vi "Calibrate_To_0.vi"(10 "Port":T2 items=["Port 1", "Port 2", "Port 3", "Port 4"], 11 "NXT":T1) -> (3 "NXT 2":T1)   [LabVIEW 2010]
uses:
  <vilib>/NXT/Subs/LVHSConnector.ctl
  <vilib>/NXT/Block Support/NXT_InputPort.ctl
  <vilib>/NXT/Dual Mode Library/Sensors/i2c_sensors.vi
panel:
  # "THIS FUNCTION WILL SIMPLY WRITE 0's TO ALL REGISTERS.\nTHIS ALLOWS MULTIPLE CALIBRATIONS WITHOUT POWERING DOWN."
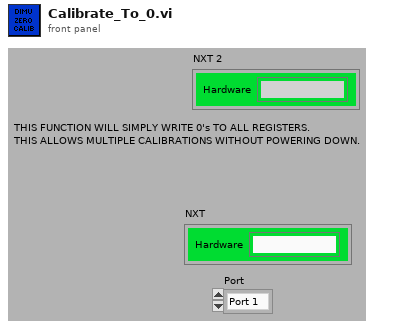
[diagram p1: front panel]
types:
  T1 = typedef "LVHSConnector.ctl" = cluster{"Hardware":string, "Flattened String":string}
  T2 = typedef "NXT_InputPort.ctl" = u8
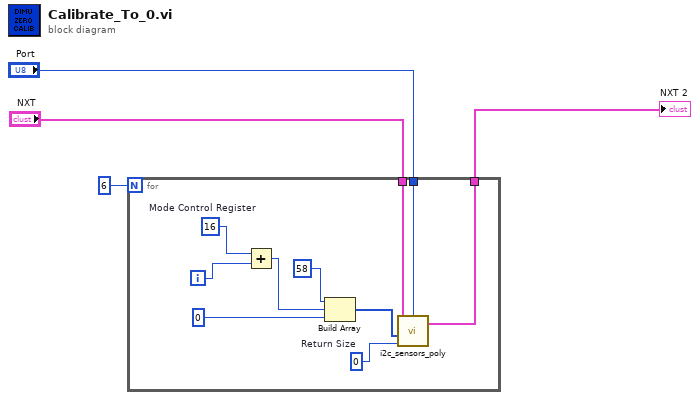
[diagram p0: block diagram]
diagram:
  n1 = for {
    N: 6 -> [_]
    tunnel: "Port" -> [w11]
    tunnel: "NXT" -> [w10]
    tunnel: [w9] -> w1
    i -> [w8]
    w13 = u8 0  # Return Size
    w7 = u8 16  # Mode Control Register
    n2 = Add(x=w7, y=w8) -> (x+y=w6:i32)
    n3 = Build Array(u8 58 ("element"), w6, 0 ("element")) -> (w14:i32[])
    n4 = call-poly <vilib>:"i2c_sensors_poly.vi"("Return Length"=w13, "Bytes to Write"=w14, "NXT"=w10, "Port"=w11) -> ("NXT"=w9:T1)  [unwired: 1 in, 2 out]
  }
  "NXT 2" <- w1
